vi "Write Flat Configuration.vi"(8 "error in (no error)":errorcluster, 10 "Configuration":variant, 11 "CIFTemplateNode in":refnum<class "CIFCorePlugin.lvclass">) -> (0 "error out":errorcluster, 3 "CIFTemplateNode out":refnum<class "CIFCorePlugin.lvclass">)   [LabVIEW 2021, in "CIFCorePlugin.lvclass"]
uses:
  CIFCorePlugin.lvclass
  CIFCorePlugin.lvclass/CIFCorePlugin.ctl
  CIFUtilities/CIFOutOfBand/CIFOutOfBand.lvclass/CIFOutOfBand.ctl
  CIFUtilities/CIFOutOfBand/Accessors/Write Local OOB Data.vi
  CIFUtilities/CIFOutOfBand/Accessors/Read Local OOB Data.vi
  CIFCoreOOB/OOB_Rx/CIFCoreOOB_Rx.lvclass
  D:/dev/CIF-LVCore/src/CIFUtilities/CIFOutOfBand/CIFOutOfBand.lvclass
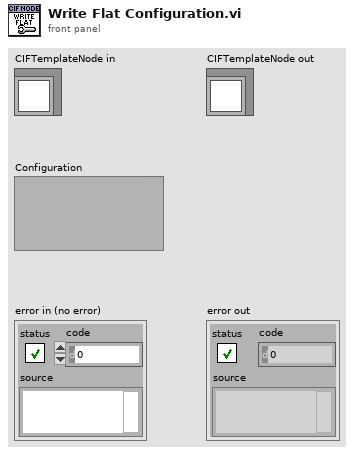
[diagram p1: front panel]
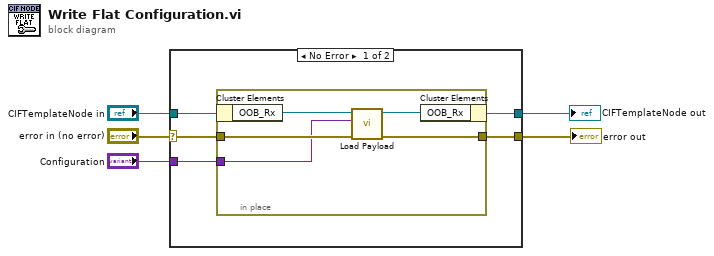
[diagram p0: block diagram]
diagram:
  n1 = case shown="No Error" "error in (no error)" {
    selector: "error in (no error)" -> [w9 w16]
    tunnel: [w8 w16] -> w4
    tunnel: [w7 w17] -> w2
    tunnel: "CIFTemplateNode in" -> [w10 w17]
    tunnel: "Configuration" -> [w6 _]
    frame No Error {
      n2 = in-place {
        in-place-border: w9 -> [w13]
        in-place-border: [w12] -> w8
        in-place-border: w6 -> [w11]
        n3 = in-place-cluster #1(w10) -> ("OOB_Rx"=w15:refnum<class "CIFCoreOOB_Rx.lvclass">)
        n4 = call "Load Payload.vi"("error in (no error)"=w13, "Configuration Payload"=w11, "CoreOOB_Rx in"=w15) -> ("error out"=w12:errorcluster, "CoreOOB_Rx out"=w14:refnum<class "CIFCoreOOB_Rx.lvclass">)  [unwired: 7 in]
        n5 = in-place-cluster #1("OOB_Rx"=w14) -> (w7:refnum<class "CIFCorePlugin.lvclass">)
      }
    }
    frame Error {
    }
  }
  "error out" <- w4
  "CIFTemplateNode out" <- w2
